vi "GameOption.vi"(11 "DataIn":T1) -> (3 "DataOut":T5)   [LabVIEW 2017]
doc: "SubVI utilizada para mostrar um pop-up para o usuário de modo que ele possa escolher qual opção de jogo deseja - Player 1 x Player 2 na mesma máquina, Player 1 x Player 2 pela rede ou Player 2 x Computador"
uses:
  controls/DataOut.ctl
  controls/Tabuleiro.ctl
  controls/GameOption.ctl
  controls/Table.ctl
  controls/DataIn.ctl
panel:
  in  "Multiplayer Remoto":bool
  in  "Difícil":bool
  in  "Fácil":bool
  in  "Médio":bool
  in  "Player 2":string
  in  "Player 1":string
  in  "Player":string
  in  "Multiplayer Local":bool
  in  "Single Player":bool
  # "Modo de Jogo"
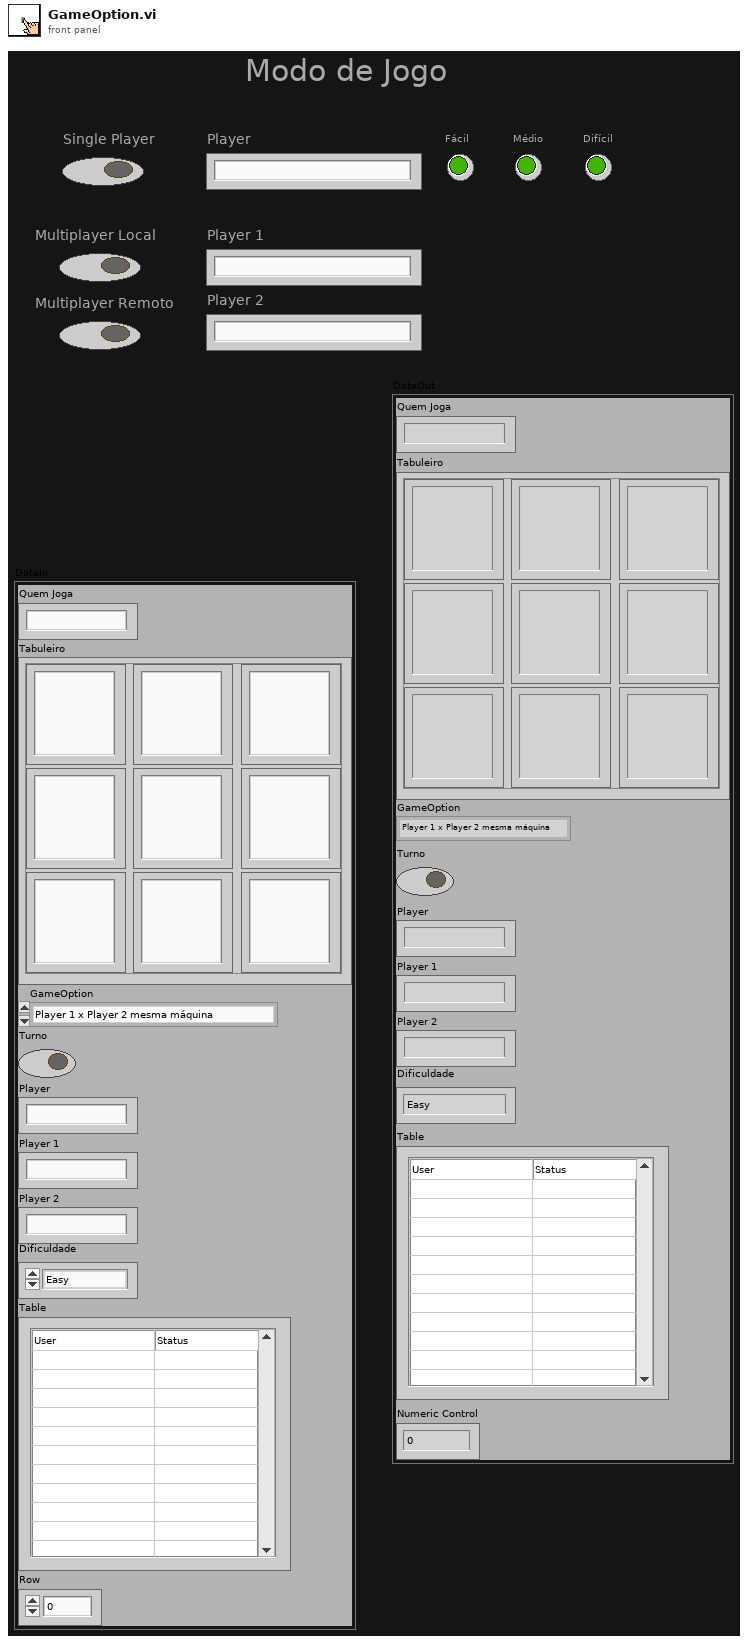
[diagram p1: front panel]
types:
  T1 = typedef "DataIn.ctl" = cluster{"Quem Joga":string, "Tabuleiro":T2, "GameOption":T3, "Turno":bool, "Player":string, "Player 1":string, "Player 2":string, "Dificuldade":enum16{"Easy", "Medium", "Hard"}, "Table":T4, "Row":u32}
  T2 = typedef "Tabuleiro.ctl" = cluster{"(0,0)":string, "(1,0)":string, "(0,1)":string, "(1,1)":string, "(2,0)":string, "(1,2)":string, "(2,2)":string, "(0,2)":string, "(2,1) ":string}
  T3 = typedef "GameOption.ctl" = enum16{"Player 1 x Player 2 mesma máquina", "Player 1 x Player 2 pela rede", "Player 1 x Computador", "Wait for Event", "Initialize", "Stop"}
  T4 = typedef "Table.ctl" = string[][]
  T5 = typedef "DataOut.ctl" = cluster{"Quem Joga":string, "Tabuleiro":T2, "GameOption":T3, "Turno":bool, "Player":string, "Player 1":string, "Player 2":string, "Dificuldade":enum16{"Easy", "Medium", "Hard"}, "Table":T4, "Numeric Control":u32}
  T6 = enum8{"Enabled", "Disabled", "Disabled and Grayed Out"}
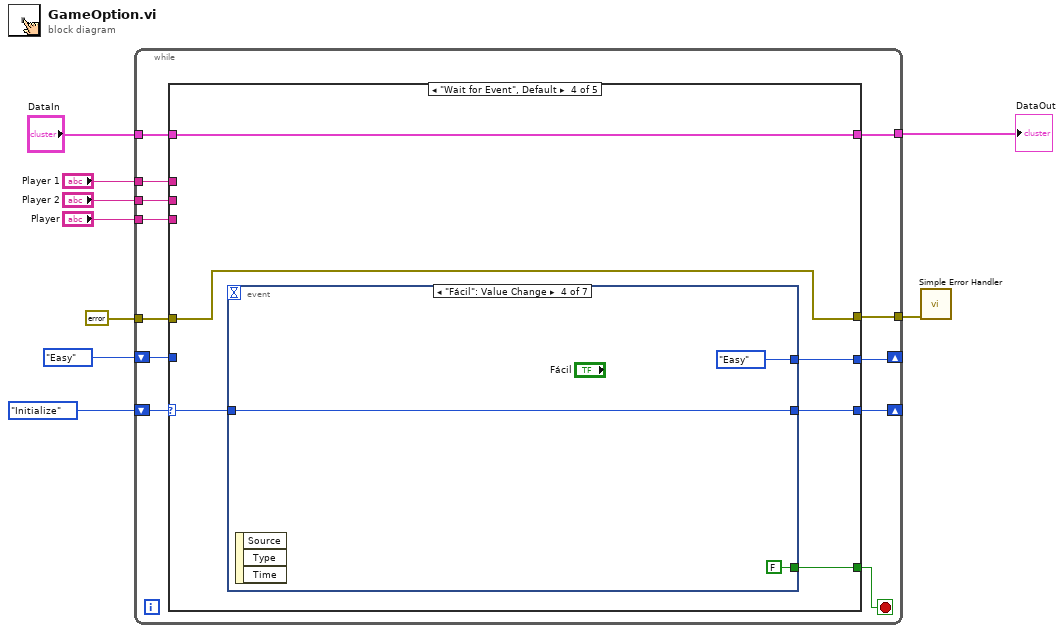
[diagram p0: block diagram]
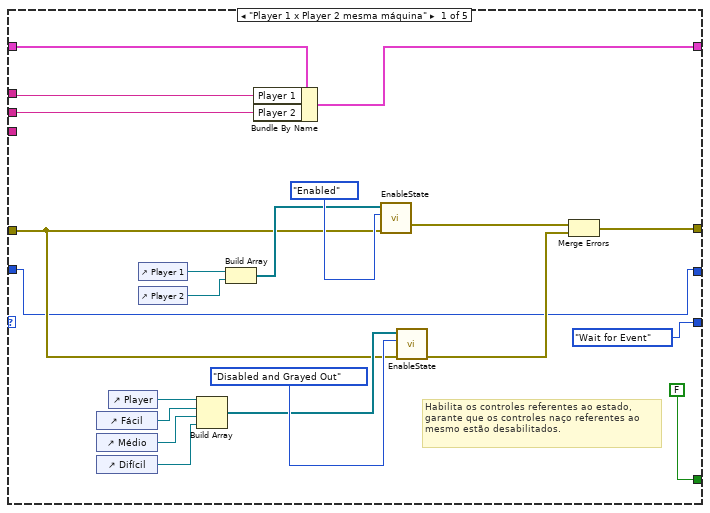
[diagram p2: hidden frame]
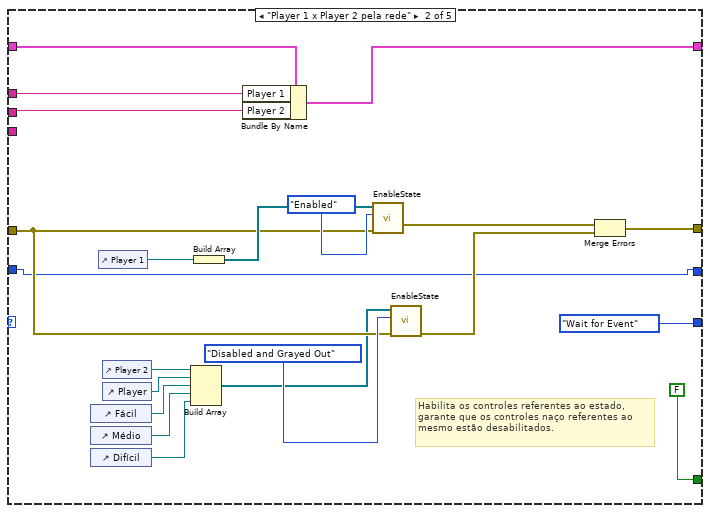
[diagram p3: hidden frame]
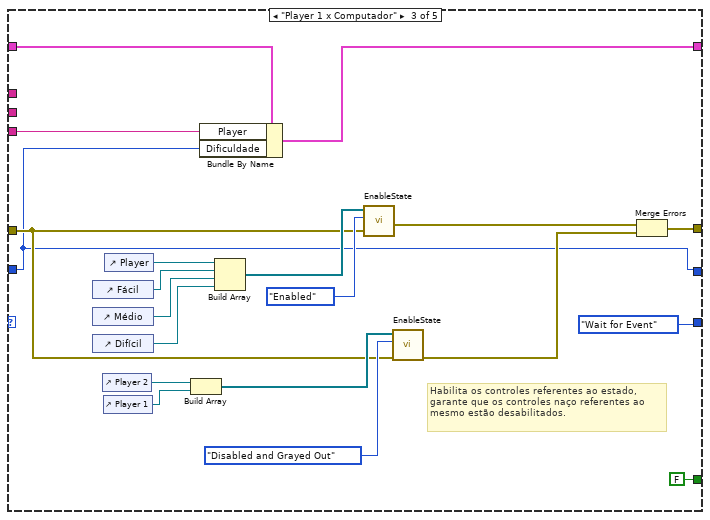
[diagram p4: hidden frame]
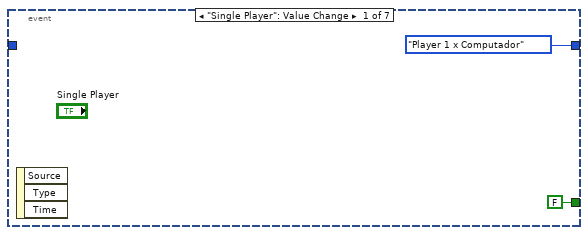
[diagram p5: hidden frame]
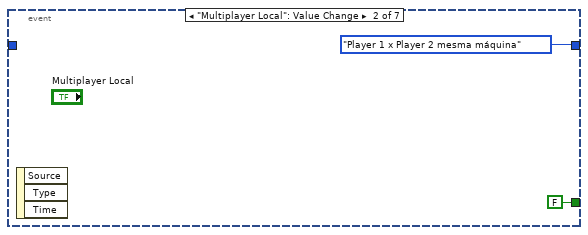
[diagram p6: hidden frame]
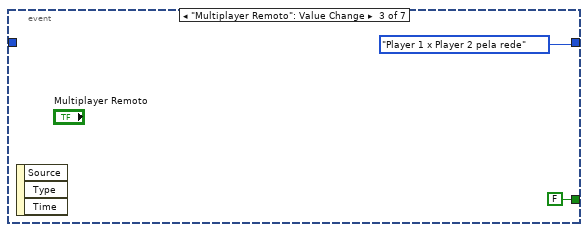
[diagram p7: hidden frame]
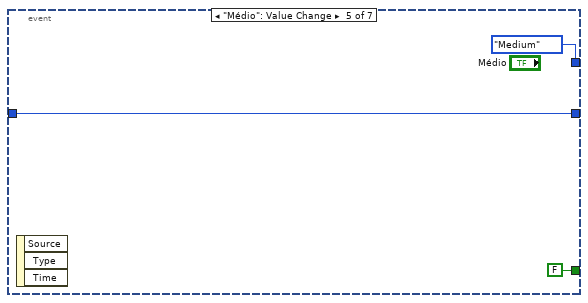
[diagram p8: hidden frame]
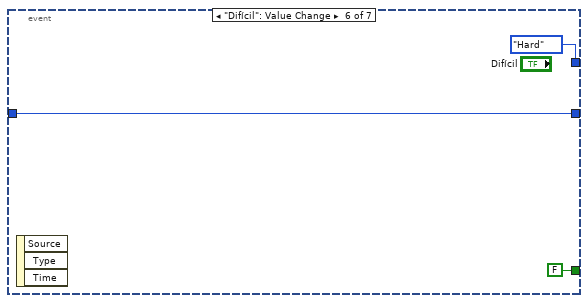
[diagram p9: hidden frame]
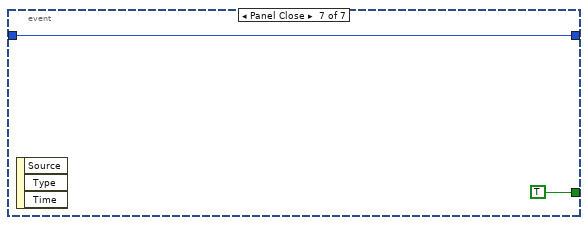
[diagram p10: hidden frame]
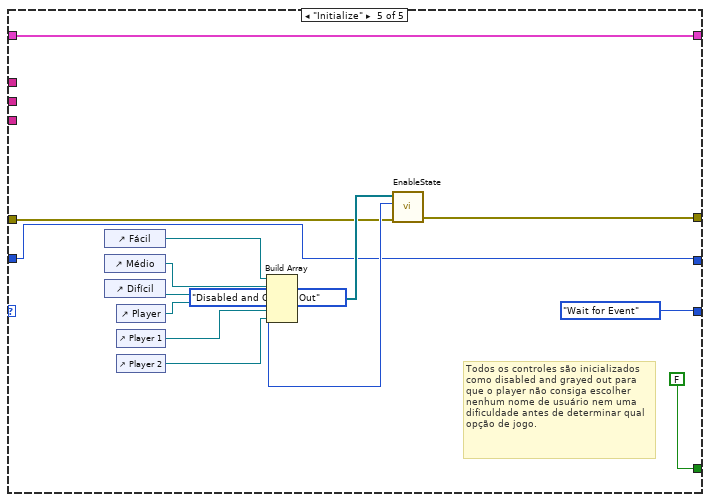
[diagram p11: hidden frame]
diagram:
  n1 = while {
    tunnel: "DataIn" -> [w21]
    shift-right: [w19] -> _
    shift-left: GameOption."Initialize" ("GameOption") -> [w20]
    tunnel: errorcluster {"status"=FALSE, "code"=0, "source"=""} ("error constant") -> [w18]
    tunnel: [w17] -> w6
    tunnel: [w15] -> w5
    tunnel: "Player 2" -> [w14]
    tunnel: "Player 1" -> [w13]
    tunnel: "Player" -> [w12]
    shift-right: [w10] -> _
    shift-left: enum16{"Easy", "Medium", "Hard"}."Easy" ("Dificuldade") -> [w11]
    stop <- w16 stop-if-true
    n2 = case shown="\"Wait for Event\", Default" w20 {
      selector: w20 -> [_ _ _ w85 _]
      tunnel: w21 -> [w26 w47 w67 w86 w108]
      tunnel: [GameOption."Wait for Event" ("GameOption") GameOption."Wait for Event" ("GameOption") GameOption."Wait for Event" ("GameOption") w89 GameOption."Wait for Event" ("GameOption")] -> w19
      tunnel: w18 -> [w31 w58 w72 w88 w111]
      tunnel: [w30 w51 w71 w88 w110] -> w17
      tunnel: [FALSE FALSE FALSE w87 FALSE] -> w16
      tunnel: [w25 w46 w66 w86 w108] -> w15
      tunnel: w14 -> [w24 w44 _ _ _]
      tunnel: w13 -> [w23 w45 _ _ _]
      tunnel: w12 -> [_ _ w65 _ _]
      tunnel: w11 -> [w22 w43 w64 _ w107]
      tunnel: [w22 w43 w64 w84 w107] -> w10
      frame "Player 1 x Player 2 mesma máquina" {
        # "Habilita os controles referentes ao estado, garante que os controles naço referentes ao mesmo estão desabilitados."
        n3 = control-ref of="Fácil"() -> (w35:refnum<vi>)
        n4 = control-ref of="Médio"() -> (w34:refnum<vi>)
        n5 = control-ref of="Difícil"() -> (w33:refnum<vi>)
        n6 = control-ref of="Player"() -> (w36:refnum<vi>)
        n7 = control-ref of="Player 1"() -> (w40:refnum<vi>)
        n8 = control-ref of="Player 2"() -> (w39:refnum<vi>)
        n9 = Build Array(w36, w35, w34, w33) -> (w32:refnum<vi>[])
        n10 = Build Array(w40, w39) -> (w38:refnum<vi>[])
        n11 = Bundle By Name(cluster=w26, "Player 1"=w23, "Player 2"=w24) -> (w25:T1)
        n12 = call "EnableState.vi"("Error In"=w31, "Disabled State"=T6."Enabled" ("Disabled"), "Controls"=w38) -> ("Error Out"=w29:errorcluster)  [unwired: 8 in]
        n13 = call "EnableState.vi"("Error In"=w31, "Disabled State"=T6."Disabled and Grayed Out" ("Disabled"), "Controls"=w32) -> ("Error Out"=w28:errorcluster)  [unwired: 8 in]
        n14 = Merge Errors(w29, w28) -> (w30:errorcluster)
      }
      frame "Player 1 x Player 2 pela rede" {
        # "Habilita os controles referentes ao estado, garante que os controles naço referentes ao mesmo estão desabilitados."
        n15 = control-ref of="Fácil"() -> (w55:refnum<vi>)
        n16 = control-ref of="Médio"() -> (w54:refnum<vi>)
        n17 = control-ref of="Difícil"() -> (w53:refnum<vi>)
        n18 = control-ref of="Player 1"() -> (w61:refnum<vi>)
        n19 = control-ref of="Player 2"() -> (w57:refnum<vi>)
        n20 = control-ref of="Player"() -> (w56:refnum<vi>)
        n21 = Build Array(w57, w56, w55, w54, w53) -> (w52:refnum<vi>[])
        n22 = Build Array(w61) -> (w60:refnum<vi>[])
        n23 = Bundle By Name(cluster=w47, "Player 1"=w45, "Player 2"=w44) -> (w46:T1)
        n24 = call "EnableState.vi"("Error In"=w58, "Disabled State"=T6."Enabled" ("Disabled"), "Controls"=w60) -> ("Error Out"=w50:errorcluster)  [unwired: 8 in]
        n25 = call "EnableState.vi"("Error In"=w58, "Disabled State"=T6."Disabled and Grayed Out" ("Disabled"), "Controls"=w52) -> ("Error Out"=w49:errorcluster)  [unwired: 8 in]
        n26 = Merge Errors(w50, w49) -> (w51:errorcluster)
      }
      frame "Player 1 x Computador" {
        # "Habilita os controles referentes ao estado, garante que os controles naço referentes ao mesmo estão desabilitados."
        n27 = control-ref of="Fácil"() -> (w80:refnum<vi>)
        n28 = control-ref of="Médio"() -> (w79:refnum<vi>)
        n29 = control-ref of="Difícil"() -> (w78:refnum<vi>)
        n30 = control-ref of="Player 2"() -> (w75:refnum<vi>)
        n31 = control-ref of="Player 1"() -> (w73:refnum<vi>)
        n32 = control-ref of="Player"() -> (w81:refnum<vi>)
        n33 = Build Array(w75, w73) -> (w74:refnum<vi>[])
        n34 = Bundle By Name(cluster=w67, "Player"=w65, "Dificuldade"=w64) -> (w66:T1)
        n35 = Build Array(w81, w80, w79, w78) -> (w77:refnum<vi>[])
        n36 = call "EnableState.vi"("Error In"=w72, "Disabled State"=T6."Enabled" ("Disabled"), "Controls"=w77) -> ("Error Out"=w70:errorcluster)  [unwired: 8 in]
        n37 = call "EnableState.vi"("Error In"=w72, "Disabled State"=T6."Disabled and Grayed Out" ("Disabled"), "Controls"=w74) -> ("Error Out"=w69:errorcluster)  [unwired: 8 in]
        n38 = Merge Errors(w70, w69) -> (w71:errorcluster)
      }
      frame "Wait for Event", Default {
        n39 = event shown="[3] \"Fácil\": Value Change" {
          selector: _ -> [_ _ _ _ _ _ _]
          dyn-events: _ -> [_ _ _ _ _ _ _]
          timeout: _ -> [_ _ _ _ _ _ _]
          tunnel: [GameOption."Player 1 x Computador" ("GameOption") GameOption."Player 1 x Player 2 mesma máquina" ("GameOption") GameOption."Player 1 x Player 2 pela rede" ("GameOption") w98 w101 w104 w105] -> w89
          tunnel: [FALSE FALSE FALSE FALSE FALSE FALSE TRUE] -> w87
          tunnel: w85 -> [_ _ _ w98 w101 w104 w105]
          tunnel: [_ _ _ enum16{"Easy", "Medium", "Hard"}."Easy" ("Dificuldade") enum16{"Easy", "Medium", "Hard"}."Medium" ("Dificuldade") enum16{"Easy", "Medium", "Hard"}."Hard" ("Dificuldade") _] -> w84
          event "Single Player": Value Change {
            n40 = event-data() -> ()  [unwired: 1 in, 3 out]
          }
          event "Multiplayer Local": Value Change {
            n41 = event-data() -> ()  [unwired: 1 in, 3 out]
          }
          event "Multiplayer Remoto": Value Change {
            n42 = event-data() -> ()  [unwired: 1 in, 3 out]
          }
          event "Fácil": Value Change {
            n43 = event-data() -> ()  [unwired: 1 in, 3 out]
          }
          event "Médio": Value Change {
            n44 = event-data() -> ()  [unwired: 1 in, 3 out]
          }
          event "Difícil": Value Change {
            n45 = event-data() -> ()  [unwired: 1 in, 3 out]
          }
          event Panel Close {
            n46 = event-data() -> ()  [unwired: 1 in, 3 out]
          }
        }
      }
      frame "Initialize" {
        # "Todos os controles são inicializados como disabled and grayed out para que o player não consiga escolher nenhum nome de usuário nem uma dificuldade antes de determinar qual opção de jogo."
        n47 = control-ref of="Fácil"() -> (w118:refnum<vi>)
        n48 = control-ref of="Médio"() -> (w117:refnum<vi>)
        n49 = control-ref of="Difícil"() -> (w116:refnum<vi>)
        n50 = control-ref of="Player"() -> (w115:refnum<vi>)
        n51 = control-ref of="Player 1"() -> (w114:refnum<vi>)
        n52 = control-ref of="Player 2"() -> (w113:refnum<vi>)
        n53 = Build Array(w118, w117, w116, w115, w114, w113) -> (w112:refnum<vi>[])
        n54 = call "EnableState.vi"("Error In"=w111, "Disabled State"=T6."Disabled and Grayed Out" ("Disabled"), "Controls"=w112) -> ("Error Out"=w110:errorcluster)  [unwired: 8 in]
      }
    }
  }
  "DataOut" <- w5
  n55 = call <vilib>:"Simple Error Handler.vi"("error in (no error)"=w6) -> ()  [unwired: 4 in, 5 out]
